vi "BRig_RT_comm_tcp_testConnect.vi"() -> ()   [LabVIEW 2014]
panel:
  out "error out":errorcluster
  in  "stop":bool
  out "Connected":bool
  out "Connecting":bool
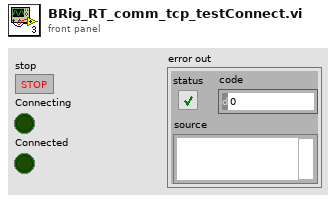
[diagram p1: front panel]
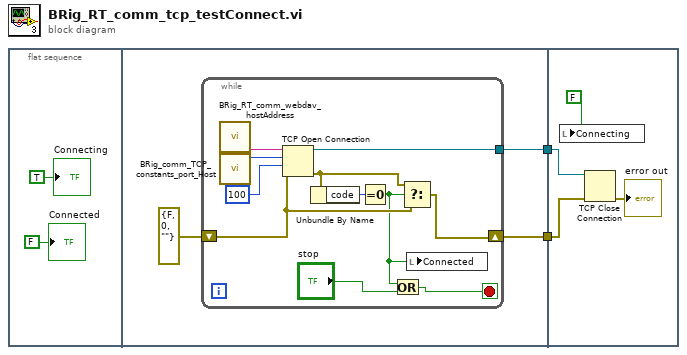
[diagram p0: block diagram]
diagram:
  n1 = flat-sequence {
    tunnel: [w6] -> w2
    tunnel: [w5] -> w1
    tunnel: w2 -> [w21]
    tunnel: w1 -> [w20]
    frame #0 {
      "Connecting" <- TRUE ("Connecting")
      "Connected" <- FALSE ("Connected")
    }
    frame #1 {
      n2 = while {
        shift-right: [w12] -> w6
        shift-left: errorcluster {"status"=FALSE, "code"=0, "source"=""} ("error in (no error)") -> [w13]
        tunnel: [w8] -> w5
        stop <- w9 stop-if-true
        n3 = call "BRig_RT_comm_webdav_hostAddress.vi"() -> ("output_HostIP"=w14:string)  [unwired: 10 in, 1 out]
        n4 = call "BRig_comm_TCP_constants_port_Host.vi"() -> ("output_TCP_port"=w15:u16)  [unwired: 11 in]
        n5 = TCP Open Connection(address=w14, remote port or service name=w15, timeout ms (60000)=100, error in (no error)=w13) -> (connection ID=w8:refnum<k5>, error out=w16:errorcluster)  [unwired: 1 in]
        n6 = Unbundle By Name(w16) -> ("code"=w17:i32)
        n7 = Equal To 0?(x=w17) -> (x = 0?=w11:bool)
        n8 = Or(x=w11, y="stop") -> (x .or. y?=w9:bool)
        n9 = Select(t=w16, s=w11, f=w13) -> (s? t:f=w12:errorcluster)
        n10 = local write "Connected"(w11) -> ()
      }
    }
    frame #2 {
      n11 = local write "Connecting"(FALSE ("Connecting")) -> ()
      n12 = TCP Close Connection(connection ID=w20, error in (no error)=w21) -> (error out=→"error out":errorcluster)  [unwired: 1 in, 1 out]
    }
  }
